vi "Get Hash Info.vi"(8 "error in (no error)":errorcluster, 11 "Hash in":refnum<class "Hash.lvclass">) -> (0 "error out":errorcluster, 1 "Output Length (Bytes)":i32, 2 "Blocksize (Bytes)":i32, 3 "Hash out":refnum<class "Hash.lvclass">)   [LabVIEW 2015, in "Crypto.lvlib" / "Hash.lvclass"]
uses:
  Hash.lvclass
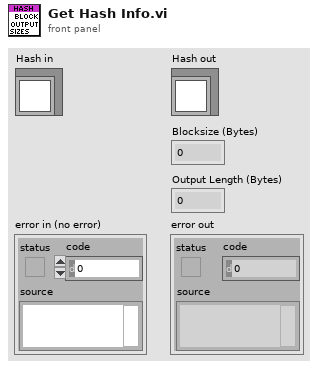
[diagram p1: front panel]
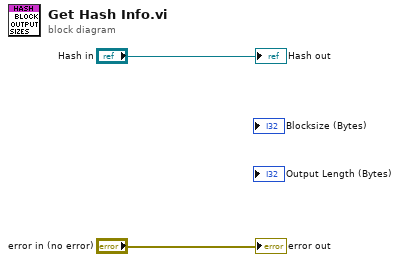
[diagram p0: block diagram]
diagram:
  "error out" <- "error in (no error)"
  "Hash out" <- "Hash in"
